vi "addBroadcastFreezeForceFrame.vi"(8 "error in (no error)":errorcluster, 9 "TriggerIRQ":bool, 10 "WaitForTrigger":bool, 11 "Subnet in":refnum<class "ISubnet.lvclass">) -> (0 "error out":errorcluster, 3 "Subnet out":refnum<class "ISubnet.lvclass">)   [LabVIEW 2015, in "ISubnet.lvclass"]
uses:
  ISubnet.lvclass
  ISubnet.lvclass/ISubnet.ctl
  Common_RT_Modbus/IModbus/IModbus.lvclass
  Common_RT_HPILC/HPILC/HPILC.lvclass
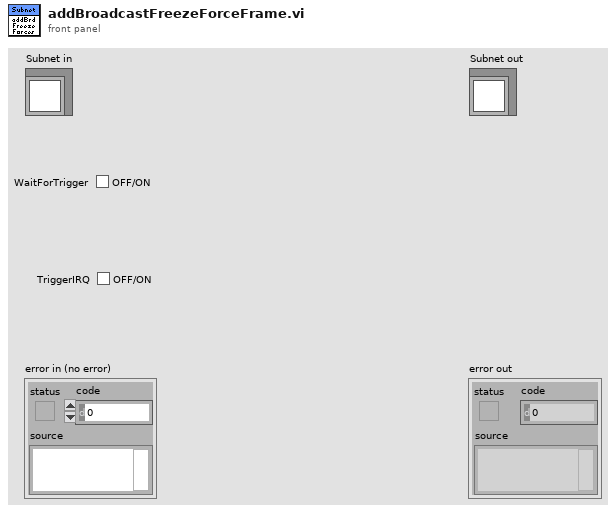
[diagram p1: front panel]
types:
  T1 = typedef "RTModbus.lvlib/Frame.ctl" = cluster{"Data":u8[], "WaitForTrigger":bool, "WaitForRx":u16, "TriggerIRQ":bool, "DelayTicks":u16, "DelayMicroseconds":u16, "DelayMilliseconds":u16}
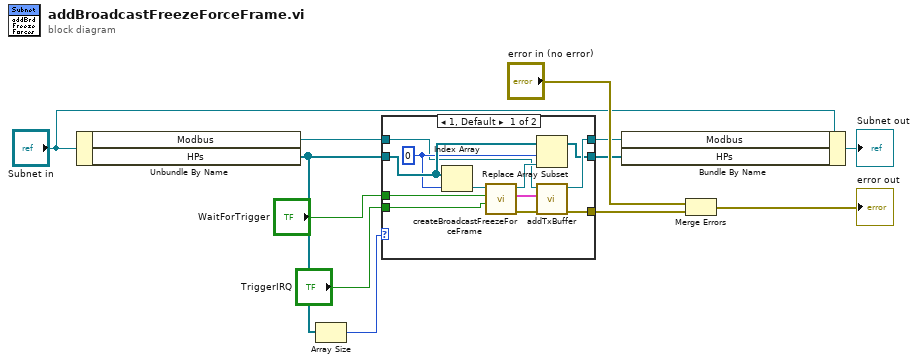
[diagram p0: block diagram]
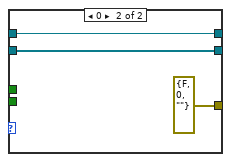
[diagram p2: hidden frame]
diagram:
  n1 = Unbundle By Name("Subnet in") -> ("Modbus"=w11:refnum<class "IModbus.lvclass">, "HPs"=w10:refnum<class "HPILC.lvclass">[])
  n2 = Array Size(array=w10) -> (size(s)=w12:i32)
  n3 = case shown="1, Default" w12 {
    tunnel: w11 -> [w20 w26]
    tunnel: w10 -> [w23 w27]
    tunnel: [w17 errorcluster {"status"=FALSE, "code"=0, "source"=""} ("error out")] -> w9
    tunnel: [w16 w26] -> w4
    tunnel: [w15 w27] -> w3
    tunnel: "WaitForTrigger" -> [w14 _]
    tunnel: "TriggerIRQ" -> [w13 _]
    frame 1, Default {
      w22 = 0 ("index")
      n4 = Index Array(array=w23, index=w22) -> (element=w24:refnum<class "HPILC.lvclass">)
      n5 = call "createBroadcastFreezeForceFrame.vi"("TriggerIRQ"=w13, "WaitForTrigger"=w14, "HardPointActuator in"=w24) -> ("error out"=w18:errorcluster, "Frame"=w19:T1, "HardPointActuator out"=w21:refnum<class "HPILC.lvclass">)  [unwired: 6 in]
      n6 = Replace Array Subset(array=w23, new element=w21, index=w22) -> (w15:refnum<class "HPILC.lvclass">[])
      n7 = call-dynamic "addTxBuffer.vi"("error in (no error)"=w18, "Frame"=w19, "IModbus in"=w20) -> ("error out"=w17:errorcluster, "IModbus out"=w16:refnum<class "IModbus.lvclass">)  [unwired: 7 in]
    }
    frame 0 {
    }
  }
  n8 = Bundle By Name(cluster="Subnet in", "Modbus"=w4, "HPs"=w3) -> (→"Subnet out":refnum<class "ISubnet.lvclass">)
  n9 = Merge Errors("error in (no error)", w9) -> (→"error out":errorcluster)
